vi "S4GUI_002.vi"(7 "Tab ObsEng":enum32{"Obs", "CCD modes", "Eng"}(tab)) -> ()   [LabVIEW 2018] (continued)
            n1451 = call-dynamic "Read mode Adm.vi"("error in (no error)"=w2493, "S4GUI in"=w2494) -> ("error out"=w2500:errorcluster, "mode Adm"=w2497:bool, "S4GUI out"=w2499:refnum<class "S4GUI.lvclass">)  [unwired: 7 in]
            n1452 = Select(t="Eng/Camera tab: password OK clicked successful" ("User Event"), s=w2497, f="Eng/Camera tab: password OK clicked with wrong input" ("User Event")) -> (s? t:f=w2498:string)
            n1453 = call-dynamic "Write User Event.vi"("error in (no error)"=w2500, "User Event"=w2498, "S4GUI in"=w2499) -> ("error out"=w2491:errorcluster, "S4GUI out"=w2492:refnum<class "S4GUI.lvclass">)  [unwired: 7 in]
          }
        }
      }
      event "enter password 2": Value Change {
        # "Verificação de senha na aba \"CCD modes\""
        n1454 = event-data() -> ("NewVal"=w2506:bool)  [unwired: 1 in]
        n1455 = case shown="True" w2506 {
          tunnel: [w2512 w2522] -> w2510
          tunnel: [w2511 w2521] -> w2509
          tunnel: w2508 -> [w2512 w2527]
          tunnel: w2507 -> [w2511 w2526]
          frame False {
          }
          frame True {
            # "Verifica senha de configuração de CCD do Administrador"
            n1456 = Equal?(x="password 2", y="ccdmodessetup") -> (x = y?=w2524:bool)
            n1457 = call-dynamic "Write mode Adm.vi"("error in (no error)"=w2526, "mode Adm"=w2524, "S4GUI in"=w2527) -> ("error out"=w2519:errorcluster, "S4GUI out"=w2520:refnum<class "S4GUI.lvclass">)  [unwired: 7 in]
            n1458 = call-dynamic "Read mode Adm.vi"("error in (no error)"=w2519, "S4GUI in"=w2520) -> ("error out"=w2517:errorcluster, "mode Adm"=w2514:bool, "S4GUI out"=w2518:refnum<class "S4GUI.lvclass">)  [unwired: 7 in]
            n1459 = Select(t="CCD mode tab: password OK clicked successful" ("User Event"), s=w2514, f="CCD mode tab: password OK clicked with wrong input" ("User Event")) -> (s? t:f=w2515:string)
            n1460 = call-dynamic "Write User Event.vi"("error in (no error)"=w2517, "User Event"=w2515, "S4GUI in"=w2518) -> ("error out"=w2521:errorcluster, "S4GUI out"=w2522:refnum<class "S4GUI.lvclass">)  [unwired: 7 in]
          }
        }
      }
      event "Tab ObsEng": Value Change {
        n1461 = event-data() -> ("NewVal"=w2528:enum32{"Obs", "CCD modes", "Eng"})  [unwired: 1 in]
        n1462 = case shown="\"CCD modes\"" w2528 {
          tunnel: [w2542 w2694 w2702] -> w2532
          tunnel: [w2544 w2692 w2701] -> w2531
          tunnel: w2530 -> [w2539 w2700 w2702]
          tunnel: w2529 -> [w2538 w2591 w2701]
          frame "CCD modes" {
            # "Sinaliza que não há requisição de SET CCD mode"
            # "Entrou na aba \"CCD modes\", ajusta para modo usuário normal..."
            n1463 = call-dynamic "Read TabAcqType index.vi"("error in (no error)"=w2538, "S4GUI in"=w2539) -> ("error out"=w2537:errorcluster, "TabAcqType index"=w2535:u32, "S4GUI out"=w2536:refnum<class "S4GUI.lvclass">)  [unwired: 7 in]
            n1464 = case shown="4" w2535 {
              tunnel: w2537 -> [w2574 w2579]
              tunnel: [w2573 w2578] -> w2540
              tunnel: [w2572 w2577] -> w2534
              tunnel: [FALSE ("Visible") TRUE ("Visible")] -> w2533
              frame 0, Default {
                n1465 = local read "Frame Transfer"() -> (w2572:enum16{"OFF", "ON"})
                n1466 = property on="Frame Transfer" class="Enum (strict)"(error in=w2574, "DisabledEnum"=T12."Enabled" ("Disabled")) -> (error out=w2573:errorcluster)  [unwired: 1 in, 1 out]
              }
              frame 4 {
                w2577 = enum16{"OFF", "ON"}."OFF" ("Frame Transfer")
                n1467 = property on="Frame Transfer" class="Enum (strict)"(error in=w2579, "DisabledEnum"=T12."Disabled and Grayed Out" ("Disabled"), "Value"=w2577) -> (error out=w2578:errorcluster)  [unwired: 1 in, 1 out]
              }
            }
            n1468 = property on="FT warning" class="Str"("Caption.Visible"=w2533) -> ()  [unwired: 2 in, 2 out]
            n1469 = call-dynamic "Write mode Adm.vi"("error in (no error)"=w2540, "mode Adm"=FALSE, "S4GUI in"=w2536) -> ("error out"=w2566:errorcluster, "S4GUI out"=w2568:refnum<class "S4GUI.lvclass">)  [unwired: 7 in]
            n1470 = local write "password 2"("" ("password")) -> ()
            n1471 = call-dynamic "Write SET request.vi"("error in (no error)"=w2566, "SET request"=FALSE, "S4GUI in"=w2568) -> ("error out"=w2565:errorcluster, "S4GUI out"=w2567:refnum<class "S4GUI.lvclass">)  [unwired: 7 in]
            n1472 = disable-structure shown="Disabled" {
              frame Disabled {
                n1473 = flat-sequence {
                  tunnel: _ -> [w2587]
                  tunnel: [w2587] -> _
                  frame #0 {
                    n1474 = local read "AQM"() -> (w2584:T4)
                    n1475 = Less Or Equal?(x=w2584, y=T4."NORMAL FAINT: Conventional; 1 MHz; Gain 2") -> (x <= y?=w2583:bool)
                    n1476 = Select(t=w2584, s=w2583, f=T4."SLOW BRIGHT: Conventional; 0.1 MHz; Gain 1" ("y")) -> (s? t:f=w2585:T4)
                    n1477 = local write "EM Gain"(u16 2 ("EM Gain")) -> ()
                    n1478 = local write "AQM"(w2585) -> ()
                  }
                }
              }
              frame Enabled {
              }
            }
            n1479 = flat-sequence {
              tunnel: w2565 -> [w2590]
              tunnel: [w2590] -> w2551
              tunnel: [w2589] -> w2548
              tunnel: [w2588] -> w2549
              frame #0 {
                w2588 = u16 2 ("EM Gain")
                w2589 = T4."NORMAL FAINT: Conventional; 1 MHz; Gain 2" ("AQM")
                n1480 = local write "EM Gain"(w2588) -> ()
                n1481 = local write "AQM"(w2589) -> ()
              }
            }
            n1482 = call-dynamic "Read CCD mode.vi"("error in (no error)"=w2551, "S4GUI in"=w2567) -> ("error out"=w2556:errorcluster, "CCD mode"=w2554:T30, "S4GUI out"=w2553:refnum<class "S4GUI.lvclass">)  [unwired: 7 in]
            n1483 = local read "SZM"() -> (w2550:T3)
            n1484 = Bundle By Name(cluster=w2554, "FTM"=w2534, "SZM"=w2550, "EM gain"=w2549, "AQM"=w2548) -> (w2555:T30)
            n1485 = call-dynamic "Write CCD mode.vi"("error in (no error)"=w2556, "CCD mode"=w2555, "S4GUI in"=w2553) -> ("error out"=w2558:errorcluster, "S4GUI out"=w2557:refnum<class "S4GUI.lvclass">)  [unwired: 7 in]
            n1486 = call-dynamic "LoadCCDmode.vi"("error in (no error)"=w2558, "S4GUI in"=w2557) -> ("error out"=w2560:errorcluster, "S4GUI out"=w2559:refnum<class "S4GUI.lvclass">)  [unwired: 8 in]
            n1487 = call-dynamic "Read Parameters CCD modes.vi"("error in (no error)"=w2560, "S4GUI in"=w2559) -> ("error out"=w2563:errorcluster, "Parameters CCD modes"=w2552:T5, "S4GUI out"=w2561:refnum<class "S4GUI.lvclass">)  [unwired: 7 in]
            n1488 = local write "Parameters CCD modes"(w2552) -> ()
            n1489 = call-dynamic "Read InfoCCDmode.vi"("error in (no error)"=w2563, "S4GUI in"=w2561) -> ("error out"=w2546:errorcluster, "InfoCCDmode"=w2562:T2, "S4GUI out"=w2547:refnum<class "S4GUI.lvclass">)  [unwired: 7 in]
            n1490 = local write "InfoCCDmode"(w2562) -> ()
            n1491 = call-dynamic "CalcTemp.vi"("error in (no error)"=w2546, "S4GUI in"=w2547) -> ("error out"=w2545:errorcluster, "S4GUI out"=w2543:refnum<class "S4GUI.lvclass">)  [unwired: 8 in]
            n1492 = call-dynamic "Read Prev Temp.vi"("error in (no error)"=w2545, "S4GUI in"=w2543) -> ("error out"=w2544:errorcluster, "Prev Temp"=w2541:dbl, "S4GUI out"=w2542:refnum<class "S4GUI.lvclass">)  [unwired: 7 in]
            n1493 = local write "Preview Temp."(w2541) -> ()
          }
          frame "Eng" {
            w2698 = T12."Disabled and Grayed Out" ("Disabled")
            # "Desabilita os botões SET."
            # "Entrou na aba  \"Eng\", ajusta para modo usuário normal..."
            n1494 = local write "password"("" ("password")) -> ()
            n1495 = call-dynamic "Write mode Adm.vi"("error in (no error)"=w2591, "mode Adm"=FALSE, "S4GUI in"=w2700) -> ("error out"=w2693:errorcluster, "S4GUI out"=w2696:refnum<class "S4GUI.lvclass">)  [unwired: 7 in]
            n1496 = property on="Set from Input ch1" class="Bool"("DisabledEnum"=w2698) -> ()  [unwired: 2 in, 2 out]
            n1497 = property on="Set from Input ch3" class="Bool"("DisabledEnum"=w2698) -> ()  [unwired: 2 in, 2 out]
            n1498 = property on="Set from Input ch2" class="Bool"("DisabledEnum"=w2698) -> ()  [unwired: 2 in, 2 out]
            n1499 = property on="Set from Input ch4" class="Bool"("DisabledEnum"=w2698) -> ()  [unwired: 2 in, 2 out]
            n1500 = local read "TARGET NAME WPSEL"() -> (w2649:enum16{"NONE", "OFF", "L/2", "L/4"})
            n1501 = call "Read Instrument.lvclass.vi"("error in (no error)"=w2693, "S4ACS_GUI in"=w2696) -> ("error out"=w2674:errorcluster, "Instrument.lvclass"=w2691:refnum<class "Instrument.lvclass">, "S4ACS_GUI out"=w2695:refnum<class "S4GUI.lvclass">)  [unwired: 7 in]
            n1502 = local read "TARGET NAME CALW"() -> (w2639:T9)
            n1503 = property on="TARGET NAME WPSEL" class="Enum (strict)"() -> ("RingText.Text"=w2647:string)  [unwired: 2 in, 2 out]
            n1504 = call "Read WPSEL.vi"("error in (no error)"=w2674, "Instrument in"=w2691) -> ("error out"=w2689:errorcluster, "Opt_Selector.lvclass"=w2687:refnum<class "Opt_Selector.lvclass">, "Instrument out"=w2690:refnum<class "Instrument.lvclass">)  [unwired: 7 in]
            n1505 = Build Array(-1.0 ("element"), 80.0 ("element"), 0.0 ("element"), 160.0 ("element")) -> (w2650:dbl[])
            n1506 = property on="TARGET NAME CALW" class="Enum (strict)"() -> ("RingText.Text"=w2638:string)  [unwired: 2 in, 2 out]
            n1507 = Build Array(-1.0 ("element"), 0.0 ("element"), 72.0 ("element"), 144.0 ("element"), 216.0 ("element"), 288.0 ("element")) -> (w2642:dbl[])
            n1508 = Index Array "Index Array"(array=w2650, index=w2649) -> (element=w2648:dbl)
            n1509 = call "Write target name.vi"("error in (no error)"=w2689, "target name"=w2647, "Optics in"=w2687) -> ("error out"=w2688:errorcluster, "Optics out"=w2686:refnum<class "Opt_Selector.lvclass">)  [unwired: 7 in]
            n1510 = Index Array(array=w2642, index=w2639) -> (element=w2637:dbl)
            n1511 = call "Write target.vi"("error in (no error)"=w2688, "target"=w2648, "Optics in"=w2686) -> ("error out"=w2684:errorcluster, "Optics out"=w2685:refnum<class "Opt_Selector.lvclass">)  [unwired: 7 in]
            n1512 = call "Write WPSEL.vi"("error in (no error)"=w2684, "Opt_Selector.lvclass"=w2685, "Instrument in"=w2690) -> ("error out"=w2683:errorcluster, "Instrument out"=w2682:refnum<class "Instrument.lvclass">)  [unwired: 7 in]
            n1513 = call "Read CALW.vi"("error in (no error)"=w2683, "Instrument in"=w2682) -> ("error out"=w2680:errorcluster, "Opt_Selector.lvclass"=w2678:refnum<class "Opt_Selector.lvclass">, "Instrument out"=w2675:refnum<class "Instrument.lvclass">)  [unwired: 7 in]
            n1514 = call "Write target name.vi"("error in (no error)"=w2680, "target name"=w2638, "Optics in"=w2678) -> ("error out"=w2681:errorcluster, "Optics out"=w2677:refnum<class "Opt_Selector.lvclass">)  [unwired: 7 in]
            n1515 = call "Write target.vi"("error in (no error)"=w2681, "target"=w2637, "Optics in"=w2677) -> ("error out"=w2679:errorcluster, "Optics out"=w2676:refnum<class "Opt_Selector.lvclass">)  [unwired: 7 in]
            n1516 = local read "TARGET NAME ASEL"() -> (w2631:enum16{"NONE", "OFF", "ON"})
            n1517 = call "Write CALW.vi"("error in (no error)"=w2679, "Opt_Selector.lvclass"=w2676, "Instrument in"=w2675) -> ("error out"=w2671:errorcluster, "Instrument out"=w2672:refnum<class "Instrument.lvclass">)  [unwired: 7 in]
            n1518 = property on="TARGET NAME ASEL" class="Enum (strict)"() -> ("RingText.Text"=w2632:string)  [unwired: 2 in, 2 out]
            n1519 = Build Array(-1.0 ("element"), 0.0 ("element"), 30.0 ("element")) -> (w2633:dbl[])
            n1520 = Index Array(array=w2633, index=w2631) -> (element=w2630:dbl)
            n1521 = call "Read ASEL.vi"("error in (no error)"=w2671, "Instrument in"=w2672) -> ("error out"=w2670:errorcluster, "Opt_Selector.lvclass"=w2668:refnum<class "Opt_Selector.lvclass">, "Instrument out"=w2665:refnum<class "Instrument.lvclass">)  [unwired: 7 in]
            n1522 = call "Write target name.vi"("error in (no error)"=w2670, "target name"=w2632, "Optics in"=w2668) -> ("error out"=w2673:errorcluster, "Optics out"=w2667:refnum<class "Opt_Selector.lvclass">)  [unwired: 7 in]
            n1523 = call "Write target.vi"("error in (no error)"=w2673, "target"=w2630, "Optics in"=w2667) -> ("error out"=w2669:errorcluster, "Optics out"=w2666:refnum<class "Opt_Selector.lvclass">)  [unwired: 7 in]
            n1524 = call "Write ASEL.vi"("error in (no error)"=w2669, "Opt_Selector.lvclass"=w2666, "Instrument in"=w2665) -> ("error out"=w2664:errorcluster, "Instrument out"=w2663:refnum<class "Instrument.lvclass">)  [unwired: 7 in]
            n1525 = local read "GMIR_target"() -> (w2624:dbl)
            n1526 = local read "GFOC_target"() -> (w2625:dbl)
            n1527 = call "Read GFOC.vi"("error in (no error)"=w2664, "Instrument in"=w2663) -> ("error out"=w2628:errorcluster, "Opt_Continuous.lvclass"=w2629:refnum<class "Opt_Continuous.lvclass">, "Instrument out"=w2660:refnum<class "Instrument.lvclass">)  [unwired: 7 in]
            n1528 = call "Write target.vi"("error in (no error)"=w2628, "target"=w2625, "Optics in"=w2629) -> ("error out"=w2662:errorcluster, "Optics out"=w2659:refnum<class "Opt_Continuous.lvclass">)  [unwired: 7 in]
            n1529 = call "Write GFOC.vi"("error in (no error)"=w2662, "Opt_Continuous.lvclass"=w2659, "Instrument in"=w2660) -> ("error out"=w2661:errorcluster, "Instrument out"=w2658:refnum<class "Instrument.lvclass">)  [unwired: 7 in]
            n1530 = call "Read GMIR.vi"("error in (no error)"=w2661, "Instrument in"=w2658) -> ("error out"=w2626:errorcluster, "Opt_Continuous.lvclass"=w2627:refnum<class "Opt_Continuous.lvclass">, "Instrument out"=w2657:refnum<class "Instrument.lvclass">)  [unwired: 7 in]
            n1531 = call "Write target.vi"("error in (no error)"=w2626, "target"=w2624, "Optics in"=w2627) -> ("error out"=w2655:errorcluster, "Optics out"=w2656:refnum<class "Opt_Continuous.lvclass">)  [unwired: 7 in]
            n1532 = local read "TARGET NAME WPROT"() -> (w2593:T10)
            n1533 = call "Write GMIR.vi"("error in (no error)"=w2655, "Opt_Continuous.lvclass"=w2656, "Instrument in"=w2657) -> ("error out"=w2620:errorcluster, "Instrument out"=w2619:refnum<class "Instrument.lvclass">)  [unwired: 7 in]
            n1534 = property on="TARGET NAME WPROT" class="Enum (strict)"() -> ("RingText.Text"=w2592:string)  [unwired: 2 in, 2 out]
            n1535 = call "Read WPROT.vi"("error in (no error)"=w2620, "Instrument in"=w2619) -> ("error out"=w2617:errorcluster, "Opt_Selector.lvclass"=w2621:refnum<class "Opt_Selector.lvclass">, "Instrument out"=w2618:refnum<class "Instrument.lvclass">)  [unwired: 7 in]
            n1536 = Build Array(-1.0 ("element"), 0.0 ("element"), 22.5 ("element"), 45.0 ("element"), 67.5 ("element"), 90.0 ("element"), 112.5 ("element"), 135.0 ("element"), 157.5 ("element"), 180.0 ("element"), 202.5 ("element"), 225.0 ("element"), 247.5 ("element"), 270.0 ("element"), 292.5 ("element"), 315.0 ("element"), 337.5 ("element")) -> (w2606:dbl[])
            n1537 = Index Array(array=w2606, index=w2593) -> (element=w2594:dbl)
            n1538 = call "Write target name.vi"("error in (no error)"=w2617, "target name"=w2592, "Optics in"=w2621) -> ("error out"=w2616:errorcluster, "Optics out"=w2623:refnum<class "Opt_Selector.lvclass">)  [unwired: 7 in]
            n1539 = call "Write target.vi"("error in (no error)"=w2616, "target"=w2594, "Optics in"=w2623) -> ("error out"=w2615:errorcluster, "Optics out"=w2622:refnum<class "Opt_Selector.lvclass">)  [unwired: 7 in]
            n1540 = call "Write WPROT.vi"("error in (no error)"=w2615, "Opt_Selector.lvclass"=w2622, "Instrument in"=w2618) -> ("error out"=w2613:errorcluster, "Instrument out"=w2614:refnum<class "Instrument.lvclass">)  [unwired: 7 in]
            n1541 = call "Write Instrument.lvclass.vi"("error in (no error)"=w2613, "Instrument.lvclass"=w2614, "S4ACS_GUI in"=w2695) -> ("error out"=w2692:errorcluster, "S4ACS_GUI out"=w2694:refnum<class "S4GUI.lvclass">)  [unwired: 7 in]
          }
          frame Default {
          }
        }
      }
      event "S4ICS protocol": Value Change {
        # "2024-04-04: Não se usa mais o ID para configurar a comunicação..."
        # "TCP-IP"
        # "ZeroMQ"
        # "Inicializar nova comunicação, de acordo\n com valor de S4ICS mode\n\nServer.Write id (T=13 ou F=5)\nInstrument.Init"
        # "Parar a comunciação atual\nServer.End"
        n1542 = event-data() -> ("NewVal"=w2705:bool)  [unwired: 1 in, 5 out]
        n1543 = call "Read Instrument.lvclass.vi"("error in (no error)"=w2715, "S4ACS_GUI in"=w2716) -> ("error out"=w2710:errorcluster, "Instrument.lvclass"=w2713:refnum<class "Instrument.lvclass">, "S4ACS_GUI out"=w2714:refnum<class "S4GUI.lvclass">)  [unwired: 7 in]
        n1544 = call-dynamic "End.vi"("error in (no error)"=w2710, "Server in"=w2713) -> ("error out"=w2709:errorcluster, "Server out"=w2712:refnum<class "Instrument.lvclass">)  [unwired: 8 in]
        n1545 = Select(t=u32 13, s=w2705, f=u32 5) -> (s? t:f=w2719:u32)
        n1546 = call-dynamic "Write id.vi"("error in (no error)"=w2709, "id"=w2719, "Server in"=w2712) -> ("error out"=w2708:errorcluster, "Server out"=w2711:refnum<class "Instrument.lvclass">)  [unwired: 7 in]
        n1547 = call-dynamic "Initialize.vi"("error in (no error)"=w2708, "Instrument in"=w2711) -> ("error out"=w2706:errorcluster, "Instrument out"=w2707:refnum<class "Instrument.lvclass">)  [unwired: 8 in]
        n1548 = call "Write Instrument.lvclass.vi"("error in (no error)"=w2706, "Instrument.lvclass"=w2707, "S4ACS_GUI in"=w2714) -> ("error out"=w2703:errorcluster, "S4ACS_GUI out"=w2704:refnum<class "S4GUI.lvclass">)  [unwired: 7 in]
      }
      event "Set from Input ch1": Value Change {
        # "ACS"
        # "GUI"
        # "EM_MODE = E.M."
        # "Readou Rate:\n30         0\n20         1     \n10         2\n1           3"
        # "EM_MODE = Conv"
        # "Readou Rate:\n1         0\n0.1      1"
        # "Readou Rate:\n1         0\n0.1      1     \n10       2\n20       3\n30       4"
        n1549 = event-data() -> ()  [unwired: 1 in, 6 out]
        n1550 = local read "Input Cluster"() -> (w2744:T8)
        n1551 = Unbundle By Name(w2744) -> ("Parameters"=w2743:T5)
        n1552 = Unbundle By Name(w2743) -> ("Image \nInitial Line"=w2771:u16, "Image\nInitial Column"=w2770:u16, "Image\nFinal Line"=w2769:u16, "Image\nFInal Column"=w2768:u16, "Vertical\nBinning"=w2767:u16, "Horizontal\nBinning"=w2766:u16, "Pre-amplification\nGain"=w2765:u8, "CCD\nEM Gain"=w2764:u16, "Readout\nRate"=w2763:u8, "Shutter\nOpenning Time"=w2762:i32, "Shutter\nClosing Time"=w2761:i32, "Vertical\nShift Speed"=w2760:u8, "Read\nMode"=w2759:u8, "Vertical\nClock Voltage"=w2758:u8, "A/D \nChannel"=w2757:u32, "Shutter\nMode"=w2756:u16, "Shutter\nTTL"=w2755:u16, "Trigger\nMode"=w2754:u16, "Frame\nTransfer"=w2735:bool, "Acquisition\nMode"=w2753:u8, "CCD \nEM Mode"=w2752:u8)
        n1553 = call-dynamic "Write User Event.vi"("error in (no error)"=w2723, "User Event"="SET CCD CONFIG CHANNEL1 ", "S4GUI in"=w2724) -> ("error out"=w2721:errorcluster, "S4GUI out"=w2722:refnum<class "S4GUI.lvclass">)  [unwired: 7 in]
        n1554 = call-dynamic "Read AcquisitionA.vi"("error in (no error)"=w2721, "S4ACS_GUI in"=w2722) -> ("error out"=w2787:errorcluster, "Acquisition.lvclass"=w2790:refnum<class "Acquisition.lvclass">, "S4ACS_GUI out"=w2791:refnum<class "S4GUI.lvclass">)  [unwired: 7 in]
        n1555 = call-dynamic "Read Channel.vi"("error in (no error)"=w2787, "Acquisition in"=w2790) -> ("error out"=w2786:errorcluster, "Channel.lvclass"=w2788:refnum<class "Channel.lvclass">, "Acquisition out"=w2789:refnum<class "Acquisition.lvclass">)  [unwired: 7 in]
        n1556 = call-dynamic "Read Interface.vi"("error in (no error)"=w2786, "Channel in"=w2788) -> ("error out"=w2734:errorcluster, "Interface.lvclass"=w2736:refnum<class "Interface.lvclass">, "Channel out"=w2731:refnum<class "Channel.lvclass">)  [unwired: 7 in]
        n1557 = call-dynamic "Write PREV_FT.vi"("error in (no error)"=w2734, "PREV_FT"=w2735, "Interface in"=w2736) -> ("error out"=w2733:errorcluster, "Interface out"=w2732:refnum<class "Interface.lvclass">)  [unwired: 7 in]
        n1558 = call-dynamic "Read target cluster.vi"("error in (no error)"=w2733, "Channel in"=w2731) -> ("error out"=w2729:errorcluster, "target cluster"=w2727:T31, "Channel out"=w2728:refnum<class "Channel.lvclass">)  [unwired: 7 in]
        n1559 = Bundle By Name(cluster=w2727, "INITIAL_LINE"=w2771, "INITIAL_COLUMN"=w2770, "FINAL_LINE"=w2769, "FINAL_COLUMN"=w2768, "VBIN"=w2767, "HBIN"=w2766, "PREAMP"=w2765, "EM_GAIN"=w2764, "READOUT_RATE"=w2763, "SHUTTER_OPENING_TIME"=w2762, "SHUTTER_CLOSING_TIME"=w2761, "VERTICAL_SHIFT_SPEED"=w2760, "READ_MODE"=w2759, "VERTICAL_CLOCK_VOLTAGE"=w2758, "AD_CHANNEL"=w2757, "SHUTTER_MODE"=w2756, "SHUTTER_TTL"=w2755, "TRIGGER_MODE"=w2754, "FRAME_TRANSFER"=w2735, "ACQUISITION_MODE"=w2753, "EM_MODE"=w2752) -> (w2726:T31)
        n1560 = call-dynamic "Write target cluster.vi"("error in (no error)"=w2729, "target cluster"=w2726, "Channel in"=w2728) -> ("error out"=w2725:errorcluster, "Channel out"=w2730:refnum<class "Channel.lvclass">)  [unwired: 7 in]
        n1561 = Flatten To String(anything=w2726, error in (no error)=w2725) -> (data string=w2775:string, error out=w2774:errorcluster)  [unwired: 2 in, 1 out]
        n1562 = call "Write flatted cluster.vi"("error in (no error)"=w2774, "flatted cluster"=w2775, "Interface in"=w2732) -> ("error out"=w2773:errorcluster, "Interface out"=w2772:refnum<class "Interface.lvclass">)  [unwired: 7 in]
        n1563 = call-dynamic "Write Interface.vi"("error in (no error)"=w2773, "Interface.lvclass"=w2772, "Channel in"=w2730) -> ("error out"=w2747:errorcluster, "Channel out"=w2750:refnum<class "Channel.lvclass">)  [unwired: 7 in]
        n1564 = call "Write section_name.vi"("error in (no error)"=w2747, "section_name"="CCD_ACS1", "Channel in"=w2750) -> ("error out"=w2746:errorcluster, "Channel out"=w2749:refnum<class "Channel.lvclass">)  [unwired: 7 in]
        n1565 = call-dynamic "save config.vi"("error in (no error)"=w2746, "file config"="lastsaved.cfg", "Channel in"=w2749) -> ("error out"=w2745:errorcluster, "Channel out"=w2748:refnum<class "Channel.lvclass">)  [unwired: 7 in]
        n1566 = call-dynamic "Read State Machine.vi"("error in (no error)"=w2745, "Device in"=w2748) -> ("error out"=w2782:errorcluster, "State Machine.lvclass"=w2784:refnum<class "State Machine.lvclass">, "Device out"=w2785:refnum<class "Channel.lvclass">)  [unwired: 7 in]
        n1567 = call-dynamic "Write State.vi"("error in (no error)"=w2782, "State"=60, "State Machine in"=w2784) -> ("error out"=w2781:errorcluster, "State Machine out"=w2783:refnum<class "State Machine.lvclass">)  [unwired: 7 in]
        n1568 = call-dynamic "Write State Machine.vi"("error in (no error)"=w2781, "State Machine.lvclass"=w2783, "Device in"=w2785) -> ("error out"=w2778:errorcluster, "Device out"=w2779:refnum<class "Channel.lvclass">)  [unwired: 7 in]
        n1569 = call-dynamic "Write Channel.vi"("error in (no error)"=w2778, "Channel.lvclass"=w2779, "Acquisition in"=w2789) -> ("error out"=w2777:errorcluster, "Acquisition out"=w2776:refnum<class "Acquisition.lvclass">)  [unwired: 7 in]
        n1570 = call-dynamic "Write AcquisitionA.vi"("error in (no error)"=w2777, "Acquisition.lvclass"=w2776, "S4ACS_GUI in"=w2791) -> ("error out"=w2738:errorcluster, "S4ACS_GUI out"=w2739:refnum<class "S4GUI.lvclass">)  [unwired: 7 in]
        n1571 = call "Write cfg file.vi"("error in (no error)"=w2738, "cfg file"="lastsaved.cfg", "S4ACS_GUI in"=w2739) -> ("error out"=w2741:errorcluster, "S4ACS_GUI out"=w2742:refnum<class "S4GUI.lvclass">)  [unwired: 7 in]
      }
      event "Input Cluster.Parameters.CCD \nEM Mode": Value Change {
        n1572 = event-data() -> ()  [unwired: 1 in, 6 out]
        n1573 = local read "Input Cluster"() -> (w2806:T8)
        n1574 = Unbundle By Name(w2806) -> ("Parameters"=w2807:T5)
        n1575 = Unbundle By Name(w2807) -> ("Readout\nRate"=→"Readout\nRate":u8, "CCD \nEM Mode"=w2801:u8)
        n1576 = case shown="0, Default" w2801 {
          tunnel: [string[] ["30 MHz", "20 MHz", "10 MHz", "1 MHz"] ("Strings []") string[] ["1 MHz", "0.1 MHz"] ("Strings []")] -> w2800
          tunnel: [u8 3 u8 0] -> w2799
          frame 0, Default {
          }
          frame 1 {
          }
        }
        n1577 = local read "Cameras Cluster"() -> (w2794:T7)
        n1578 = flat-sequence {
          tunnel: w2799 -> [w2809]
          tunnel: w2800 -> [w2808]
          tunnel: w2801 -> [w2810]
          tunnel: [w2810] -> w2798
          tunnel: [w2809] -> w2796
          tunnel: w2807 -> [w2816]
          tunnel: [w2815] -> w2805
          tunnel: w2798 -> [w2811]
          tunnel: w2796 -> [w2812]
          tunnel: w2795 -> [w2814]
          tunnel: [w2813] -> w2793
          frame #0 {
            n1579 = property on="Readout\nRate" class="Ring (strict)"("Strings []"=w2808) -> ()  [unwired: 2 in, 2 out]
            n1580 = property on="Readout Rate" class="Ring (strict)"("Strings []"=w2808) -> ()  [unwired: 2 in, 2 out]
            n1581 = property on="Readout Rate 4" class="Ring (strict)"("Strings []"=w2808) -> ()  [unwired: 2 in, 2 out]
            n1582 = property on="Readout Rate 2" class="Ring (strict)"("Strings []"=w2808) -> ()  [unwired: 2 in, 2 out]
            n1583 = property on="Readout Rate 3" class="Ring (strict)"("Strings []"=w2808) -> ()  [unwired: 2 in, 2 out]
          }
          frame #1 {
            n1584 = Bundle By Name(cluster=w2814, "Readout Rate"=w2812, "Read Mode"=w2811) -> (w2813:T32)
            n1585 = Bundle By Name(cluster=w2816, "Readout\nRate"=w2812, "CCD \nEM Mode"=w2811) -> (w2815:T5)
          }
        }
        n1586 = Unbundle By Name(w2794) -> ("Current Configuration"=w2795:T32)
        n1587 = Bundle By Name(cluster=w2806, "Parameters"=w2805) -> (w2804:T8)
        n1588 = local write "Input Cluster"(w2804) -> ()
        n1589 = Bundle By Name(cluster=w2794, "Current Configuration"=w2793) -> (w2792:T7)
        n1590 = local write "Cameras Cluster"(w2792) -> ()
      }
      event "Set from Input ch2": Value Change {
        n1591 = event-data() -> ()  [unwired: 1 in, 6 out]
        n1592 = local read "Input Cluster"() -> (w2845:T8)
        n1593 = Unbundle By Name(w2845) -> ("Parameters"=w2844:T5)
        n1594 = call-dynamic "Write User Event.vi"("error in (no error)"=w2823, "User Event"="SET CCD CONFIG CHANNEL2 ", "S4GUI in"=w2824) -> ("error out"=w2821:errorcluster, "S4GUI out"=w2822:refnum<class "S4GUI.lvclass">)  [unwired: 7 in]
        n1595 = Unbundle By Name(w2844) -> ("Image \nInitial Line"=w2872:u16, "Image\nInitial Column"=w2871:u16, "Image\nFinal Line"=w2870:u16, "Image\nFInal Column"=w2869:u16, "Vertical\nBinning"=w2868:u16, "Horizontal\nBinning"=w2867:u16, "Pre-amplification\nGain"=w2866:u8, "CCD\nEM Gain"=w2865:u16, "Readout\nRate"=w2864:u8, "Shutter\nOpenning Time"=w2863:i32, "Shutter\nClosing Time"=w2862:i32, "Vertical\nShift Speed"=w2861:u8, "Read\nMode"=w2860:u8, "Vertical\nClock Voltage"=w2859:u8, "A/D \nChannel"=w2858:u32, "Shutter\nMode"=w2857:u16, "Shutter\nTTL"=w2856:u16, "Trigger\nMode"=w2855:u16, "Frame\nTransfer"=w2835:bool, "Acquisition\nMode"=w2854:u8, "CCD \nEM Mode"=w2853:u8)
        n1596 = call "Read AcquisitionB.vi"("error in (no error)"=w2821, "S4ACS_GUI in"=w2822) -> ("error out"=w2888:errorcluster, "Acquisition.lvclass"=w2891:refnum<class "Acquisition.lvclass">, "S4ACS_GUI out"=w2892:refnum<class "S4GUI.lvclass">)  [unwired: 7 in]
        n1597 = call-dynamic "Read Channel.vi"("error in (no error)"=w2888, "Acquisition in"=w2891) -> ("error out"=w2887:errorcluster, "Channel.lvclass"=w2889:refnum<class "Channel.lvclass">, "Acquisition out"=w2890:refnum<class "Acquisition.lvclass">)  [unwired: 7 in]
        n1598 = call-dynamic "Read Interface.vi"("error in (no error)"=w2887, "Channel in"=w2889) -> ("error out"=w2836:errorcluster, "Interface.lvclass"=w2837:refnum<class "Interface.lvclass">, "Channel out"=w2832:refnum<class "Channel.lvclass">)  [unwired: 7 in]
        n1599 = call-dynamic "Write PREV_FT.vi"("error in (no error)"=w2836, "PREV_FT"=w2835, "Interface in"=w2837) -> ("error out"=w2829:errorcluster, "Interface out"=w2827:refnum<class "Interface.lvclass">)  [unwired: 7 in]
        n1600 = call-dynamic "Read target cluster.vi"("error in (no error)"=w2829, "Channel in"=w2832) -> ("error out"=w2834:errorcluster, "target cluster"=w2831:T31, "Channel out"=w2833:refnum<class "Channel.lvclass">)  [unwired: 7 in]
        n1601 = Bundle By Name(cluster=w2831, "INITIAL_LINE"=w2872, "INITIAL_COLUMN"=w2871, "FINAL_LINE"=w2870, "FINAL_COLUMN"=w2869, "VBIN"=w2868, "HBIN"=w2867, "PREAMP"=w2866, "EM_GAIN"=w2865, "READOUT_RATE"=w2864, "SHUTTER_OPENING_TIME"=w2863, "SHUTTER_CLOSING_TIME"=w2862, "VERTICAL_SHIFT_SPEED"=w2861, "READ_MODE"=w2860, "VERTICAL_CLOCK_VOLTAGE"=w2859, "AD_CHANNEL"=w2858, "SHUTTER_MODE"=w2857, "SHUTTER_TTL"=w2856, "TRIGGER_MODE"=w2855, "FRAME_TRANSFER"=w2835, "ACQUISITION_MODE"=w2854, "EM_MODE"=w2853) -> (w2830:T31)
        n1602 = call-dynamic "Write target cluster.vi"("error in (no error)"=w2834, "target cluster"=w2830, "Channel in"=w2833) -> ("error out"=w2828:errorcluster, "Channel out"=w2826:refnum<class "Channel.lvclass">)  [unwired: 7 in]
        n1603 = Flatten To String(anything=w2830, error in (no error)=w2828) -> (data string=w2876:string, error out=w2875:errorcluster)  [unwired: 2 in, 1 out]
        n1604 = call "Write flatted cluster.vi"("error in (no error)"=w2875, "flatted cluster"=w2876, "Interface in"=w2827) -> ("error out"=w2874:errorcluster, "Interface out"=w2873:refnum<class "Interface.lvclass">)  [unwired: 7 in]
        n1605 = call-dynamic "Write Interface.vi"("error in (no error)"=w2874, "Interface.lvclass"=w2873, "Channel in"=w2826) -> ("error out"=w2848:errorcluster, "Channel out"=w2851:refnum<class "Channel.lvclass">)  [unwired: 7 in]
        n1606 = call "Write section_name.vi"("error in (no error)"=w2848, "section_name"="CCD_ACS2", "Channel in"=w2851) -> ("error out"=w2847:errorcluster, "Channel out"=w2850:refnum<class "Channel.lvclass">)  [unwired: 7 in]
        n1607 = call-dynamic "save config.vi"("error in (no error)"=w2847, "file config"="lastsaved.cfg", "Channel in"=w2850) -> ("error out"=w2846:errorcluster, "Channel out"=w2849:refnum<class "Channel.lvclass">)  [unwired: 7 in]
        n1608 = call-dynamic "Read State Machine.vi"("error in (no error)"=w2846, "Device in"=w2849) -> ("error out"=w2883:errorcluster, "State Machine.lvclass"=w2885:refnum<class "State Machine.lvclass">, "Device out"=w2886:refnum<class "Channel.lvclass">)  [unwired: 7 in]
        n1609 = call-dynamic "Write State.vi"("error in (no error)"=w2883, "State"=60, "State Machine in"=w2885) -> ("error out"=w2882:errorcluster, "State Machine out"=w2884:refnum<class "State Machine.lvclass">)  [unwired: 7 in]
        n1610 = call-dynamic "Write State Machine.vi"("error in (no error)"=w2882, "State Machine.lvclass"=w2884, "Device in"=w2886) -> ("error out"=w2879:errorcluster, "Device out"=w2880:refnum<class "Channel.lvclass">)  [unwired: 7 in]
        n1611 = call-dynamic "Write Channel.vi"("error in (no error)"=w2879, "Channel.lvclass"=w2880, "Acquisition in"=w2890) -> ("error out"=w2878:errorcluster, "Acquisition out"=w2877:refnum<class "Acquisition.lvclass">)  [unwired: 7 in]
        n1612 = call "Write AcquisitionB.vi"("error in (no error)"=w2878, "Acquisition.lvclass"=w2877, "S4ACS_GUI in"=w2892) -> ("error out"=w2838:errorcluster, "S4ACS_GUI out"=w2839:refnum<class "S4GUI.lvclass">)  [unwired: 7 in]
        n1613 = call "Write cfg file.vi"("error in (no error)"=w2838, "cfg file"="lastsaved.cfg", "S4ACS_GUI in"=w2839) -> ("error out"=w2841:errorcluster, "S4ACS_GUI out"=w2842:refnum<class "S4GUI.lvclass">)  [unwired: 7 in]
      }
      event "Set from Input ch3": Value Change {
        n1614 = event-data() -> ()  [unwired: 1 in, 6 out]
        n1615 = local read "Input Cluster"() -> (w2917:T8)
        n1616 = Unbundle By Name(w2917) -> ("Parameters"=w2916:T5)
        n1617 = call-dynamic "Write User Event.vi"("error in (no error)"=w2895, "User Event"="SET CCD CONFIG CHANNEL 3 ", "S4GUI in"=w2896) -> ("error out"=w2893:errorcluster, "S4GUI out"=w2894:refnum<class "S4GUI.lvclass">)  [unwired: 7 in]
        n1618 = Unbundle By Name(w2916) -> ("Image \nInitial Line"=w2944:u16, "Image\nInitial Column"=w2943:u16, "Image\nFinal Line"=w2942:u16, "Image\nFInal Column"=w2941:u16, "Vertical\nBinning"=w2940:u16, "Horizontal\nBinning"=w2939:u16, "Pre-amplification\nGain"=w2938:u8, "CCD\nEM Gain"=w2937:u16, "Readout\nRate"=w2936:u8, "Shutter\nOpenning Time"=w2935:i32, "Shutter\nClosing Time"=w2934:i32, "Vertical\nShift Speed"=w2933:u8, "Read\nMode"=w2932:u8, "Vertical\nClock Voltage"=w2931:u8, "A/D \nChannel"=w2930:u32, "Shutter\nMode"=w2929:u16, "Shutter\nTTL"=w2928:u16, "Trigger\nMode"=w2927:u16, "Frame\nTransfer"=w2907:bool, "Acquisition\nMode"=w2926:u8, "CCD \nEM Mode"=w2925:u8)
        n1619 = call-dynamic "Read AcquisitionC.vi"("error in (no error)"=w2893, "S4ACS_GUI in"=w2894) -> ("error out"=w2960:errorcluster, "Acquisition.lvclass"=w2963:refnum<class "Acquisition.lvclass">, "S4ACS_GUI out"=w2964:refnum<class "S4GUI.lvclass">)  [unwired: 7 in]
        n1620 = call-dynamic "Read Channel.vi"("error in (no error)"=w2960, "Acquisition in"=w2963) -> ("error out"=w2959:errorcluster, "Channel.lvclass"=w2961:refnum<class "Channel.lvclass">, "Acquisition out"=w2962:refnum<class "Acquisition.lvclass">)  [unwired: 7 in]
        n1621 = call-dynamic "Read Interface.vi"("error in (no error)"=w2959, "Channel in"=w2961) -> ("error out"=w2908:errorcluster, "Interface.lvclass"=w2909:refnum<class "Interface.lvclass">, "Channel out"=w2904:refnum<class "Channel.lvclass">)  [unwired: 7 in]
        n1622 = call-dynamic "Write PREV_FT.vi"("error in (no error)"=w2908, "PREV_FT"=w2907, "Interface in"=w2909) -> ("error out"=w2898:errorcluster, "Interface out"=w2905:refnum<class "Interface.lvclass">)  [unwired: 7 in]
        n1623 = call-dynamic "Read target cluster.vi"("error in (no error)"=w2898, "Channel in"=w2904) -> ("error out"=w2906:errorcluster, "target cluster"=w2900:T31, "Channel out"=w2903:refnum<class "Channel.lvclass">)  [unwired: 7 in]
        n1624 = Bundle By Name(cluster=w2900, "INITIAL_LINE"=w2944, "INITIAL_COLUMN"=w2943, "FINAL_LINE"=w2942, "FINAL_COLUMN"=w2941, "VBIN"=w2940, "HBIN"=w2939, "PREAMP"=w2938, "EM_GAIN"=w2937, "READOUT_RATE"=w2936, "SHUTTER_OPENING_TIME"=w2935, "SHUTTER_CLOSING_TIME"=w2934, "VERTICAL_SHIFT_SPEED"=w2933, "READ_MODE"=w2932, "VERTICAL_CLOCK_VOLTAGE"=w2931, "AD_CHANNEL"=w2930, "SHUTTER_MODE"=w2929, "SHUTTER_TTL"=w2928, "TRIGGER_MODE"=w2927, "FRAME_TRANSFER"=w2907, "ACQUISITION_MODE"=w2926, "EM_MODE"=w2925) -> (w2899:T31)
        n1625 = call-dynamic "Write target cluster.vi"("error in (no error)"=w2906, "target cluster"=w2899, "Channel in"=w2903) -> ("error out"=w2901:errorcluster, "Channel out"=w2902:refnum<class "Channel.lvclass">)  [unwired: 7 in]
        n1626 = Flatten To String(anything=w2899, error in (no error)=w2901) -> (data string=w2948:string, error out=w2947:errorcluster)  [unwired: 2 in, 1 out]
        n1627 = call "Write flatted cluster.vi"("error in (no error)"=w2947, "flatted cluster"=w2948, "Interface in"=w2905) -> ("error out"=w2946:errorcluster, "Interface out"=w2945:refnum<class "Interface.lvclass">)  [unwired: 7 in]
        n1628 = call-dynamic "Write Interface.vi"("error in (no error)"=w2946, "Interface.lvclass"=w2945, "Channel in"=w2902) -> ("error out"=w2920:errorcluster, "Channel out"=w2923:refnum<class "Channel.lvclass">)  [unwired: 7 in]
        n1629 = call "Write section_name.vi"("error in (no error)"=w2920, "section_name"="CCD_ACS3", "Channel in"=w2923) -> ("error out"=w2919:errorcluster, "Channel out"=w2922:refnum<class "Channel.lvclass">)  [unwired: 7 in]
        n1630 = call-dynamic "save config.vi"("error in (no error)"=w2919, "file config"="lastsaved.cfg", "Channel in"=w2922) -> ("error out"=w2918:errorcluster, "Channel out"=w2921:refnum<class "Channel.lvclass">)  [unwired: 7 in]
        n1631 = call-dynamic "Read State Machine.vi"("error in (no error)"=w2918, "Device in"=w2921) -> ("error out"=w2955:errorcluster, "State Machine.lvclass"=w2957:refnum<class "State Machine.lvclass">, "Device out"=w2958:refnum<class "Channel.lvclass">)  [unwired: 7 in]
        n1632 = call-dynamic "Write State.vi"("error in (no error)"=w2955, "State"=60, "State Machine in"=w2957) -> ("error out"=w2954:errorcluster, "State Machine out"=w2956:refnum<class "State Machine.lvclass">)  [unwired: 7 in]
        n1633 = call-dynamic "Write State Machine.vi"("error in (no error)"=w2954, "State Machine.lvclass"=w2956, "Device in"=w2958) -> ("error out"=w2951:errorcluster, "Device out"=w2952:refnum<class "Channel.lvclass">)  [unwired: 7 in]
        n1634 = call-dynamic "Write Channel.vi"("error in (no error)"=w2951, "Channel.lvclass"=w2952, "Acquisition in"=w2962) -> ("error out"=w2950:errorcluster, "Acquisition out"=w2949:refnum<class "Acquisition.lvclass">)  [unwired: 7 in]
        n1635 = call-dynamic "Write AcquisitionC.vi"("error in (no error)"=w2950, "Acquisition.lvclass"=w2949, "S4ACS_GUI in"=w2964) -> ("error out"=w2910:errorcluster, "S4ACS_GUI out"=w2911:refnum<class "S4GUI.lvclass">)  [unwired: 7 in]
        n1636 = call "Write cfg file.vi"("error in (no error)"=w2910, "cfg file"="lastsaved.cfg", "S4ACS_GUI in"=w2911) -> ("error out"=w2913:errorcluster, "S4ACS_GUI out"=w2914:refnum<class "S4GUI.lvclass">)  [unwired: 7 in]
      }
      event "Set from Input ch4": Value Change {
        n1637 = event-data() -> ()  [unwired: 1 in, 6 out]
        n1638 = local read "Input Cluster"() -> (w2989:T8)
        n1639 = Unbundle By Name(w2989) -> ("Parameters"=w2988:T5)
        n1640 = call-dynamic "Write User Event.vi"("error in (no error)"=w2968, "User Event"="SET CCD CONFIG CHANNEL4 ", "S4GUI in"=w2967) -> ("error out"=w2965:errorcluster, "S4GUI out"=w2966:refnum<class "S4GUI.lvclass">)  [unwired: 7 in]
        n1641 = Unbundle By Name(w2988) -> ("Image \nInitial Line"=w3016:u16, "Image\nInitial Column"=w3015:u16, "Image\nFinal Line"=w3014:u16, "Image\nFInal Column"=w3013:u16, "Vertical\nBinning"=w3012:u16, "Horizontal\nBinning"=w3011:u16, "Pre-amplification\nGain"=w3010:u8, "CCD\nEM Gain"=w3009:u16, "Readout\nRate"=w3008:u8, "Shutter\nOpenning Time"=w3007:i32, "Shutter\nClosing Time"=w3006:i32, "Vertical\nShift Speed"=w3005:u8, "Read\nMode"=w3004:u8, "Vertical\nClock Voltage"=w3003:u8, "A/D \nChannel"=w3002:u32, "Shutter\nMode"=w3001:u16, "Shutter\nTTL"=w3000:u16, "Trigger\nMode"=w2999:u16, "Frame\nTransfer"=w2979:bool, "Acquisition\nMode"=w2998:u8, "CCD \nEM Mode"=w2997:u8)
        n1642 = call-dynamic "Read AcquisitionD.vi"("error in (no error)"=w2965, "S4ACS_GUI in"=w2966) -> ("error out"=w3032:errorcluster, "Acquisition.lvclass"=w3035:refnum<class "Acquisition.lvclass">, "S4ACS_GUI out"=w3036:refnum<class "S4GUI.lvclass">)  [unwired: 7 in]
        n1643 = call-dynamic "Read Channel.vi"("error in (no error)"=w3032, "Acquisition in"=w3035) -> ("error out"=w3031:errorcluster, "Channel.lvclass"=w3033:refnum<class "Channel.lvclass">, "Acquisition out"=w3034:refnum<class "Acquisition.lvclass">)  [unwired: 7 in]
        n1644 = call-dynamic "Read Interface.vi"("error in (no error)"=w3031, "Channel in"=w3033) -> ("error out"=w2980:errorcluster, "Interface.lvclass"=w2981:refnum<class "Interface.lvclass">, "Channel out"=w2976:refnum<class "Channel.lvclass">)  [unwired: 7 in]
        n1645 = call-dynamic "Write PREV_FT.vi"("error in (no error)"=w2980, "PREV_FT"=w2979, "Interface in"=w2981) -> ("error out"=w2971:errorcluster, "Interface out"=w2977:refnum<class "Interface.lvclass">)  [unwired: 7 in]
        n1646 = call-dynamic "Read target cluster.vi"("error in (no error)"=w2971, "Channel in"=w2976) -> ("error out"=w2978:errorcluster, "target cluster"=w2975:T31, "Channel out"=w2974:refnum<class "Channel.lvclass">)  [unwired: 7 in]
        n1647 = Bundle By Name(cluster=w2975, "INITIAL_LINE"=w3016, "INITIAL_COLUMN"=w3015, "FINAL_LINE"=w3014, "FINAL_COLUMN"=w3013, "VBIN"=w3012, "HBIN"=w3011, "PREAMP"=w3010, "EM_GAIN"=w3009, "READOUT_RATE"=w3008, "SHUTTER_OPENING_TIME"=w3007, "SHUTTER_CLOSING_TIME"=w3006, "VERTICAL_SHIFT_SPEED"=w3005, "READ_MODE"=w3004, "VERTICAL_CLOCK_VOLTAGE"=w3003, "AD_CHANNEL"=w3002, "SHUTTER_MODE"=w3001, "SHUTTER_TTL"=w3000, "TRIGGER_MODE"=w2999, "FRAME_TRANSFER"=w2979, "ACQUISITION_MODE"=w2998, "EM_MODE"=w2997) -> (w2973:T31)
        n1648 = call-dynamic "Write target cluster.vi"("error in (no error)"=w2978, "target cluster"=w2973, "Channel in"=w2974) -> ("error out"=w2972:errorcluster, "Channel out"=w2970:refnum<class "Channel.lvclass">)  [unwired: 7 in]
        n1649 = Flatten To String(anything=w2973, error in (no error)=w2972) -> (data string=w3020:string, error out=w3019:errorcluster)  [unwired: 2 in, 1 out]
        n1650 = call "Write flatted cluster.vi"("error in (no error)"=w3019, "flatted cluster"=w3020, "Interface in"=w2977) -> ("error out"=w3018:errorcluster, "Interface out"=w3017:refnum<class "Interface.lvclass">)  [unwired: 7 in]
        n1651 = call-dynamic "Write Interface.vi"("error in (no error)"=w3018, "Interface.lvclass"=w3017, "Channel in"=w2970) -> ("error out"=w2992:errorcluster, "Channel out"=w2995:refnum<class "Channel.lvclass">)  [unwired: 7 in]
        n1652 = call "Write section_name.vi"("error in (no error)"=w2992, "section_name"="CCD_ACS4", "Channel in"=w2995) -> ("error out"=w2991:errorcluster, "Channel out"=w2994:refnum<class "Channel.lvclass">)  [unwired: 7 in]
        n1653 = call-dynamic "save config.vi"("error in (no error)"=w2991, "file config"="lastsaved.cfg", "Channel in"=w2994) -> ("error out"=w2990:errorcluster, "Channel out"=w2993:refnum<class "Channel.lvclass">)  [unwired: 7 in]
        n1654 = call-dynamic "Read State Machine.vi"("error in (no error)"=w2990, "Device in"=w2993) -> ("error out"=w3027:errorcluster, "State Machine.lvclass"=w3029:refnum<class "State Machine.lvclass">, "Device out"=w3030:refnum<class "Channel.lvclass">)  [unwired: 7 in]
        n1655 = call-dynamic "Write State.vi"("error in (no error)"=w3027, "State"=60, "State Machine in"=w3029) -> ("error out"=w3026:errorcluster, "State Machine out"=w3028:refnum<class "State Machine.lvclass">)  [unwired: 7 in]
        n1656 = call-dynamic "Write State Machine.vi"("error in (no error)"=w3026, "State Machine.lvclass"=w3028, "Device in"=w3030) -> ("error out"=w3023:errorcluster, "Device out"=w3024:refnum<class "Channel.lvclass">)  [unwired: 7 in]
        n1657 = call-dynamic "Write Channel.vi"("error in (no error)"=w3023, "Channel.lvclass"=w3024, "Acquisition in"=w3034) -> ("error out"=w3022:errorcluster, "Acquisition out"=w3021:refnum<class "Acquisition.lvclass">)  [unwired: 7 in]
        n1658 = call-dynamic "Write AcquisitionD.vi"("error in (no error)"=w3022, "Acquisition.lvclass"=w3021, "S4ACS_GUI in"=w3036) -> ("error out"=w2982:errorcluster, "S4ACS_GUI out"=w2983:refnum<class "S4GUI.lvclass">)  [unwired: 7 in]
        n1659 = call "Write cfg file.vi"("error in (no error)"=w2982, "cfg file"="lastsaved.cfg", "S4ACS_GUI in"=w2983) -> ("error out"=w2985:errorcluster, "S4ACS_GUI out"=w2986:refnum<class "S4GUI.lvclass">)  [unwired: 7 in]
      }
      event "Restore Default ch1": Value Change {
        n1660 = event-data() -> ()  [unwired: 1 in, 6 out]
        n1661 = call-dynamic "Read AcquisitionA.vi"("error in (no error)"=w3067, "S4ACS_GUI in"=w3068) -> ("error out"=w3063:errorcluster, "Acquisition.lvclass"=w3065:refnum<class "Acquisition.lvclass">, "S4ACS_GUI out"=w3066:refnum<class "S4GUI.lvclass">)  [unwired: 7 in]
        n1662 = call-dynamic "Read Channel.vi"("error in (no error)"=w3063, "Acquisition in"=w3065) -> ("error out"=w3050:errorcluster, "Channel.lvclass"=w3052:refnum<class "Channel.lvclass">, "Acquisition out"=w3064:refnum<class "Acquisition.lvclass">)  [unwired: 7 in]
        n1663 = call "Write section_name.vi"("error in (no error)"=w3050, "section_name"="CCD_ACS1", "Channel in"=w3052) -> ("error out"=w3049:errorcluster, "Channel out"=w3051:refnum<class "Channel.lvclass">)  [unwired: 7 in]
        n1664 = call-dynamic "load config.vi"("error in (no error)"=w3049, "cfg file name"="default.cfg", "Channel in"=w3051) -> ("error out"=w3047:errorcluster, "Channel out"=w3048:refnum<class "Channel.lvclass">)  [unwired: 7 in]
        n1665 = call-dynamic "Read State Machine.vi"("error in (no error)"=w3047, "Device in"=w3048) -> ("error out"=w3059:errorcluster, "State Machine.lvclass"=w3061:refnum<class "State Machine.lvclass">, "Device out"=w3062:refnum<class "Channel.lvclass">)  [unwired: 7 in]
        n1666 = call-dynamic "Write State.vi"("error in (no error)"=w3059, "State"=60, "State Machine in"=w3061) -> ("error out"=w3058:errorcluster, "State Machine out"=w3060:refnum<class "State Machine.lvclass">)  [unwired: 7 in]
        n1667 = call-dynamic "Write State Machine.vi"("error in (no error)"=w3058, "State Machine.lvclass"=w3060, "Device in"=w3062) -> ("error out"=w3043:errorcluster, "Device out"=w3039:refnum<class "Channel.lvclass">)  [unwired: 7 in]
        n1668 = call "Write section_name.vi"("error in (no error)"=w3043, "section_name"="CCD_ACS1", "Channel in"=w3039) -> ("error out"=w3044:errorcluster, "Channel out"=w3038:refnum<class "Channel.lvclass">)  [unwired: 7 in]
        n1669 = call-dynamic "save config.vi"("error in (no error)"=w3044, "file config"="lastsaved.cfg", "Channel in"=w3038) -> ("error out"=w3042:errorcluster, "Channel out"=w3037:refnum<class "Channel.lvclass">)  [unwired: 7 in]
        n1670 = call-dynamic "Write Channel.vi"("error in (no error)"=w3042, "Channel.lvclass"=w3037, "Acquisition in"=w3064) -> ("error out"=w3056:errorcluster, "Acquisition out"=w3055:refnum<class "Acquisition.lvclass">)  [unwired: 7 in]
        n1671 = call-dynamic "Write AcquisitionA.vi"("error in (no error)"=w3056, "Acquisition.lvclass"=w3055, "S4ACS_GUI in"=w3066) -> ("error out"=w3054:errorcluster, "S4ACS_GUI out"=w3045:refnum<class "S4GUI.lvclass">)  [unwired: 7 in]
      }
      event "Load Button": Value Change {
        (unwired) "C:\\Users\\observer\\sparc4\\s4gui\\Config" ("default name")
        n1672 = event-data() -> ()  [unwired: 1 in, 6 out]
        n1673 = String To Path(string="D:\\sparc4\\config\\s4gui" ("default name")) -> (path=w3072:path)
        n1674 = call "File Dialog"("start path"=w3072, "prompt"="Select file...", "button label"="Open", "default name"="lastsaved.cfg", "error in"=w3074, "pattern (all files)"="*.cfg") -> ("selected path"=w3071:path, "cancelled"=w3075:bool, "error out"=→"error out 2":errorcluster)  [unwired: 6 in, 1 out]
        n1675 = Strip Path(path=w3071) -> (name=w3070:string)  [unwired: 1 out]
        n1676 = case shown="False" w3075 {
          tunnel: w3082 -> [w3215 w3217]
          tunnel: [w3131 w3217] -> w3081
          tunnel: [w3129 w3216] -> w3080
          tunnel: w3074 -> [w3128 w3216]
          tunnel: w3070 -> [w3127 _]
          frame False {
            n1677 = call-dynamic "Read AcquisitionA.vi"("error in (no error)"=w3128, "S4ACS_GUI in"=w3215) -> ("error out"=w3211:errorcluster, "Acquisition.lvclass"=w3213:refnum<class "Acquisition.lvclass">, "S4ACS_GUI out"=w3214:refnum<class "S4GUI.lvclass">)  [unwired: 7 in]
            n1678 = call-dynamic "Read Channel.vi"("error in (no error)"=w3211, "Acquisition in"=w3213) -> ("error out"=w3198:errorcluster, "Channel.lvclass"=w3200:refnum<class "Channel.lvclass">, "Acquisition out"=w3212:refnum<class "Acquisition.lvclass">)  [unwired: 7 in]
            n1679 = call "Write section_name.vi"("error in (no error)"=w3198, "section_name"="CCD_ACS1", "Channel in"=w3200) -> ("error out"=w3197:errorcluster, "Channel out"=w3199:refnum<class "Channel.lvclass">)  [unwired: 7 in]
            n1680 = call-dynamic "load config.vi"("error in (no error)"=w3197, "cfg file name"=w3127, "Channel in"=w3199) -> ("error out"=w3125:errorcluster, "Channel out"=w3126:refnum<class "Channel.lvclass">)  [unwired: 7 in]
            n1681 = call-dynamic "save config.vi"("error in (no error)"=w3125, "file config"="lastsaved.cfg", "Channel in"=w3126) -> ("error out"=w3107:errorcluster, "Channel out"=w3108:refnum<class "Channel.lvclass">)  [unwired: 7 in]
            n1682 = call-dynamic "Read target cluster.vi"("error in (no error)"=w3107, "Channel in"=w3108) -> ("target cluster"=w3083:T31)  [unwired: 7 in, 2 out]
            n1683 = call-dynamic "Read State Machine.vi"("error in (no error)"=w3107, "Device in"=w3108) -> ("error out"=w3207:errorcluster, "State Machine.lvclass"=w3209:refnum<class "State Machine.lvclass">, "Device out"=w3210:refnum<class "Channel.lvclass">)  [unwired: 7 in]
            n1684 = call-dynamic "Write State.vi"("error in (no error)"=w3207, "State"=60, "State Machine in"=w3209) -> ("error out"=w3206:errorcluster, "State Machine out"=w3208:refnum<class "State Machine.lvclass">)  [unwired: 7 in]
            n1685 = call-dynamic "Write State Machine.vi"("error in (no error)"=w3206, "State Machine.lvclass"=w3208, "Device in"=w3210) -> ("error out"=w3203:errorcluster, "Device out"=w3204:refnum<class "Channel.lvclass">)  [unwired: 7 in]
            n1686 = call-dynamic "Write Channel.vi"("error in (no error)"=w3203, "Channel.lvclass"=w3204, "Acquisition in"=w3212) -> ("error out"=w3202:errorcluster, "Acquisition out"=w3201:refnum<class "Acquisition.lvclass">)  [unwired: 7 in]
            n1687 = call-dynamic "Write AcquisitionA.vi"("error in (no error)"=w3202, "Acquisition.lvclass"=w3201, "S4ACS_GUI in"=w3214) -> ("error out"=w3138:errorcluster, "S4ACS_GUI out"=w3137:refnum<class "S4GUI.lvclass">)  [unwired: 7 in]
            n1688 = call "Read AcquisitionB.vi"("error in (no error)"=w3138, "S4ACS_GUI in"=w3137) -> ("error out"=w3180:errorcluster, "Acquisition.lvclass"=w3178:refnum<class "Acquisition.lvclass">, "S4ACS_GUI out"=w3177:refnum<class "S4GUI.lvclass">)  [unwired: 7 in]
            n1689 = call-dynamic "Read Channel.vi"("error in (no error)"=w3180, "Acquisition in"=w3178) -> ("error out"=w3193:errorcluster, "Channel.lvclass"=w3191:refnum<class "Channel.lvclass">, "Acquisition out"=w3179:refnum<class "Acquisition.lvclass">)  [unwired: 7 in]
            n1690 = call "Write section_name.vi"("error in (no error)"=w3193, "section_name"="CCD_ACS2", "Channel in"=w3191) -> ("error out"=w3194:errorcluster, "Channel out"=w3192:refnum<class "Channel.lvclass">)  [unwired: 7 in]
            n1691 = call-dynamic "load config.vi"("error in (no error)"=w3194, "cfg file name"=w3127, "Channel in"=w3192) -> ("error out"=w3122:errorcluster, "Channel out"=w3120:refnum<class "Channel.lvclass">)  [unwired: 7 in]
            n1692 = call-dynamic "save config.vi"("error in (no error)"=w3122, "file config"="lastsaved.cfg", "Channel in"=w3120) -> ("error out"=w3121:errorcluster, "Channel out"=w3119:refnum<class "Channel.lvclass">)  [unwired: 7 in]
            n1693 = call-dynamic "Read State Machine.vi"("error in (no error)"=w3121, "Device in"=w3119) -> ("error out"=w3184:errorcluster, "State Machine.lvclass"=w3182:refnum<class "State Machine.lvclass">, "Device out"=w3181:refnum<class "Channel.lvclass">)  [unwired: 7 in]
            n1694 = call-dynamic "Write State.vi"("error in (no error)"=w3184, "State"=60, "State Machine in"=w3182) -> ("error out"=w3185:errorcluster, "State Machine out"=w3183:refnum<class "State Machine.lvclass">)  [unwired: 7 in]
            n1695 = call-dynamic "Write State Machine.vi"("error in (no error)"=w3185, "State Machine.lvclass"=w3183, "Device in"=w3181) -> ("error out"=w3188:errorcluster, "Device out"=w3187:refnum<class "Channel.lvclass">)  [unwired: 7 in]
            n1696 = call-dynamic "Write Channel.vi"("error in (no error)"=w3188, "Channel.lvclass"=w3187, "Acquisition in"=w3179) -> ("error out"=w3189:errorcluster, "Acquisition out"=w3190:refnum<class "Acquisition.lvclass">)  [unwired: 7 in]
